vi "new_document.vi"(0 "Device In":T1, 1 "Name In":string, 11 "error in":errorcluster) -> (3 "Comm":T2, 4 "Device Out":T1, 15 "error out":errorcluster)   [LabVIEW 2019]
uses:
  <userlib>/IoT Devices/_subVIs/HTTPComm.ctl
panel:
  out "id":string
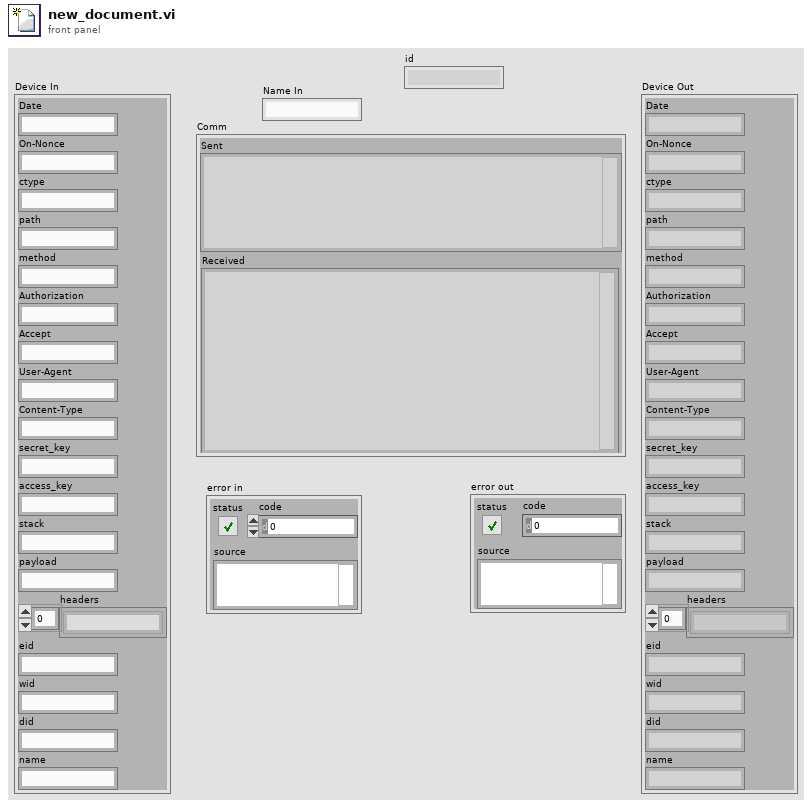
[diagram p1: front panel]
types:
  T1 = cluster{"Date":string, "On-Nonce":string, "ctype":string, "path":string, "method":string, "Authorization":string, "Accept":string, "User-Agent":string, "Content-Type":string, "secret_key":string, "access_key":string, "stack":string, "payload":string, "headers":string[], "eid":string, "wid":string, "did":string, "name":string}
  T2 = typedef "HTTPComm.ctl" = cluster{"url":string, "sent headers":string, "sent body":string, "headers":string, "body":string, "Sent":string, "Received":string}
  T3 = cluster{"name":string, "defaultWorkspace":cluster{"documentId":string, "id":string}}
  T4 = cluster{"name":string, "ownerType":i32, "isPublic":bool}
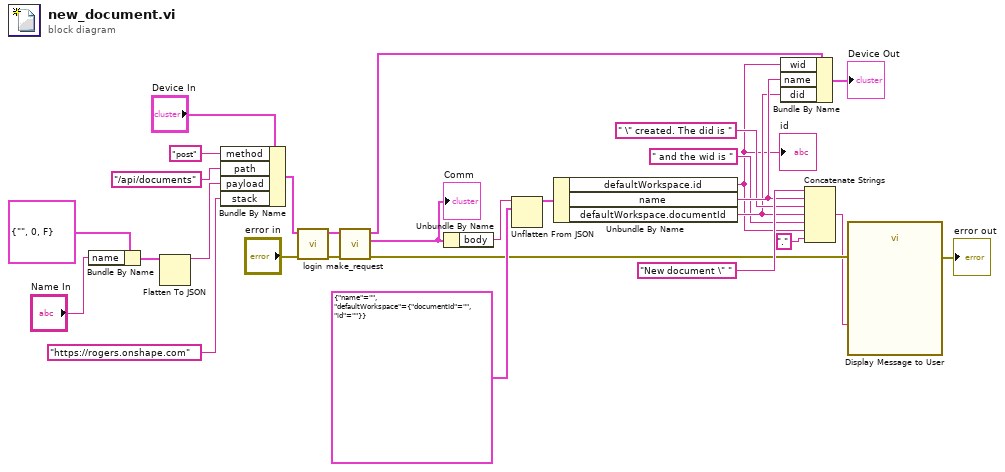
[diagram p0: block diagram]
diagram:
  n1 = Bundle By Name(cluster=T4 {"name"="", "ownerType"=0, "isPublic"=FALSE}, "name"="Name In") -> (w27:T4)
  n2 = Flatten To JSON(anything=w27) -> (JSON string=w23:string)  [unwired: 2 in, 1 out]
  n3 = Bundle By Name(cluster="Device In", "method"="post" ("Method"), "path"="/api/documents" ("payload"), "payload"=w23, "stack"="https://rogers.onshape.com" ("stacks")) -> (w14:T1)
  n4 = call <userlib>:"login.vi"("error in"="error in", "Device In"=w14) -> ("error out"=w11:errorcluster, "Device Out"=w13:T1)  [unwired: 8 in]
  n5 = call <userlib>:"make_request.vi"("Error in"=w11, "Device In"=w13) -> ("error out"=w3:errorcluster, "Comm"=w20:T2, "Device Out"=w16:T1)  [unwired: 7 in]
  "Comm" <- w20
  n6 = Unbundle By Name(w20) -> ("body"=w19:string)
  n7 = Unflatten From JSON(JSON string=w19, type and defaults=T3 {"name"="", "defaultWorkspace"={"documentId"="", "id"=""}}) -> (value=w17:T3)  [unwired: 5 in, 1 out]
  n8 = Unbundle By Name(w17) -> ("defaultWorkspace.id"=w5:string, "name"=w9:string, "defaultWorkspace.documentId"=w7:string)
  "id" <- w5
  n9 = Bundle By Name(cluster=w16, "wid"=w5, "name"=w9, "did"=w7) -> (→"Device Out":T1)
  n10 = Concatenate Strings("New document \" " ("string"), w9, " \" created. The did is " ("string"), w7, " and the wid is " ("string"), w5, "." ("string")) -> (w1:string)
  n11 = call "Display Message to User"("error in (no error)"=w3, "Message"=w1) -> ("error out"=→"error out":errorcluster)  [unwired: 8 in, 1 out]
